vi "ArrayCharToString.vi"(7 "Type":T1(ring), 11 "TAB":string[][](array[string])) -> (3 "Instruction":string)   [LabVIEW 2020]
doc: "Convert array data to string instruction for script python"
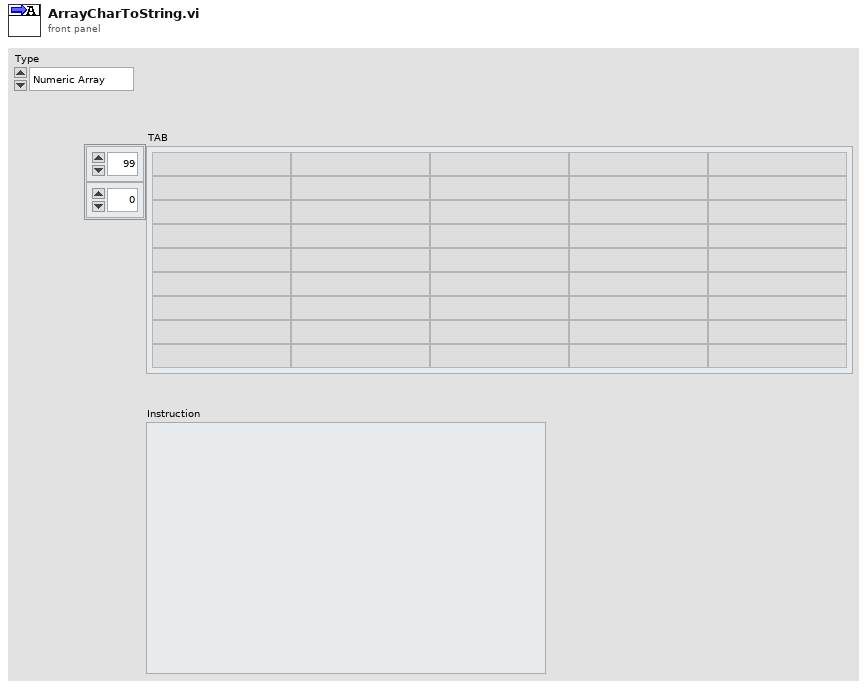
[diagram p1: front panel]
types:
  T1 = enum16{"Numeric Array", "String Array", "Sparse"}
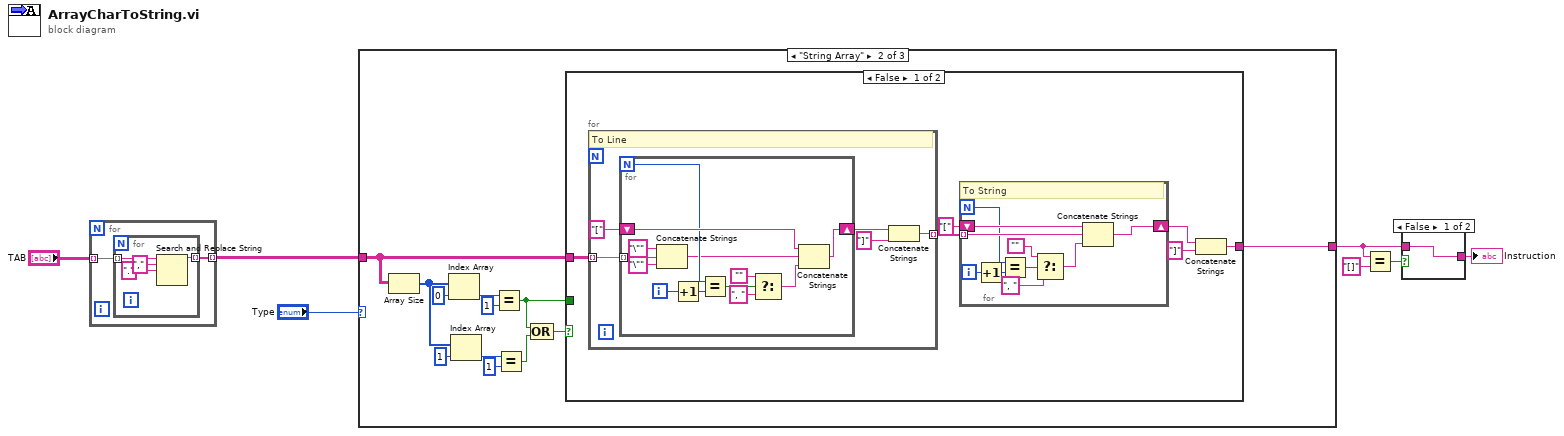
[diagram p0: block diagram]
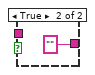
[diagram p2: hidden frame]
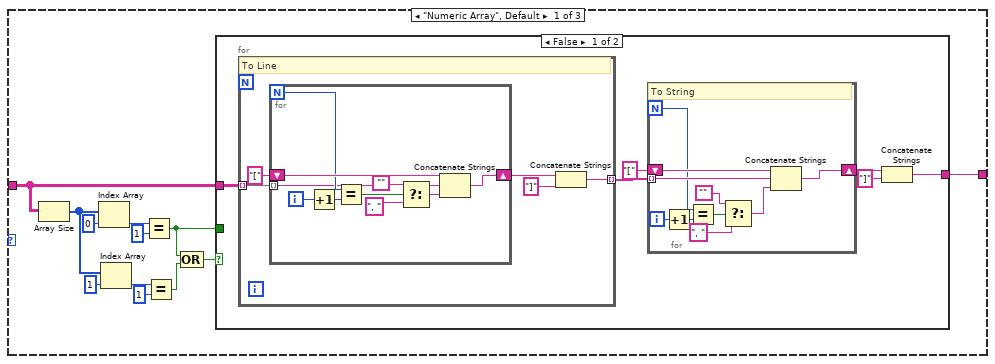
[diagram p3: hidden frame]
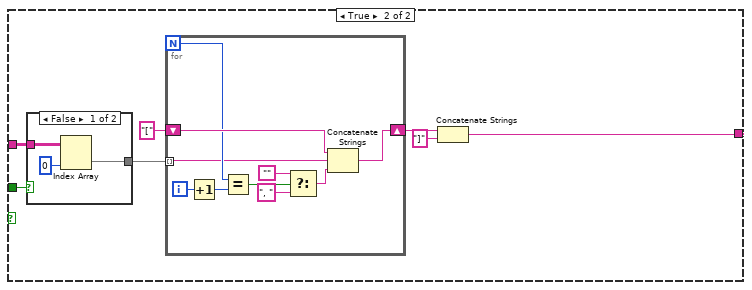
[diagram p4: hidden frame]
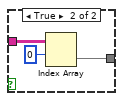
[diagram p5: hidden frame]
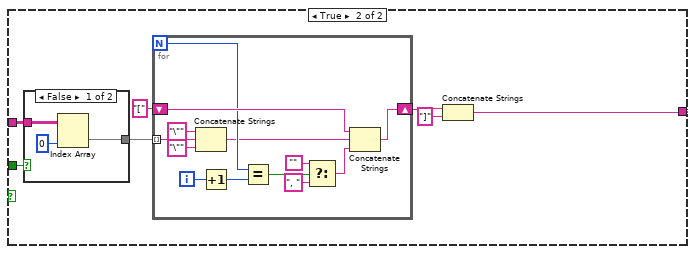
[diagram p6: hidden frame]
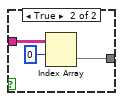
[diagram p7: hidden frame]
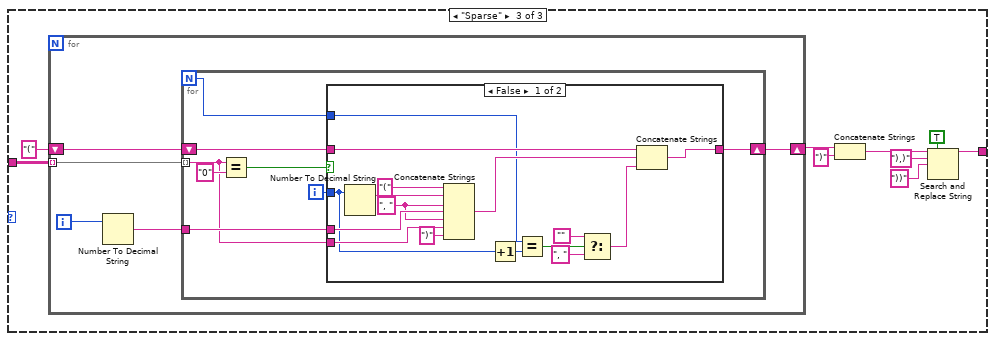
[diagram p8: hidden frame]
diagram:
  n1 = for {
    tunnel: "TAB" -> [w9] mode=indexing
    tunnel: [w8] -> w2 mode=indexing
    n2 = for {
      tunnel: w9 -> [w13] mode=indexing
      tunnel: [w10] -> w8 mode=indexing
      n3 = Search and Replace String(input string=w13, search string=",", replace string="." ("replace string (\"\")")) -> (result string=w10:string)  [unwired: 5 in, 3 out]
    }
  }
  n4 = case shown="\"String Array\"" "Type" {
    tunnel: w2 -> [w25 w91 w160]
    tunnel: [w22 w88 w155] -> w4
    frame "Numeric Array", Default {
      n5 = Array Size(array=w25) -> (size(s)=w20:i32[])
      n6 = Index Array(array=w20, index=0) -> (element=w19:i32)
      n7 = Index Array(array=w20, index=1) -> (element=w17:i32)
      n8 = Equal?(x=w19, y=1) -> (x = y?=w14:bool)
      n9 = Equal?(x=w17, y=1) -> (x = y?=w16:bool)
      n10 = Compound Arithmetic op=OR(w14, w16) -> (w15:bool)
      n11 = case shown="False" w15 {
        tunnel: [w27 w58] -> w22
        tunnel: w25 -> [w26 w60]
        tunnel: w14 -> [_ w57]
        frame False {
          n12 = for {
            tunnel: w26 -> [w46] mode=indexing
            tunnel: [w44] -> w31 mode=indexing
            # "To Line"
            n13 = for {
              N -> [w53]
              shift-right: [w55] -> w45
              shift-left: "[" ("t") -> [w56]
              tunnel: w46 -> [w47] mode=indexing
              i -> [w54]
              n14 = Increment(x=w54) -> (x+1=w52:i32)
              n15 = Equal?(x=w53, y=w52) -> (x = y?=w51:bool)
              n16 = Select(t="", s=w51, f=", ") -> (s? t:f=w49:string)
              n17 = Concatenate Strings(w56, w47, w49) -> (w55:string)
            }
            n18 = Concatenate Strings(w45, "]" ("t")) -> (w44:string)
          }
          n19 = for {
            N -> [w37]
            shift-right: [w39] -> w29
            shift-left: "[" -> [w41]
            tunnel: w31 -> [w40] mode=indexing
            i -> [w38]
            # "To String"
            n20 = Increment(x=w38) -> (x+1=w36:i32)
            n21 = Equal?(x=w37, y=w36) -> (x = y?=w35:bool)
            n22 = Select(t="", s=w35, f=", ") -> (s? t:f=w33:string)
            n23 = Concatenate Strings(w41, w40, w33) -> (w39:string)
          }
          n24 = Concatenate Strings(w29, "]" ("string")) -> (w27:string)
        }
        frame True {
          n25 = case shown="False" w57 {
            tunnel: w60 -> [w66 w69]
            tunnel: [w65 w68] -> w59
            frame False {
              n26 = Index Array(array=w66, index (col)=0 ("disabled index (col)")) -> (element=w65:string[])  [unwired: 1 in]
            }
            frame True {
              n27 = Index Array(array=w69, index (row)=0) -> (element=w68:string[])  [unwired: 1 in]
            }
          }
          n28 = for {
            N -> [w73]
            tunnel: w59 -> [w71] mode=indexing
            shift-right: [w70] -> w62
            shift-left: "[" -> [w79]
            i -> [w74]
            n29 = Increment(x=w74) -> (x+1=w78:i32)
            n30 = Equal?(x=w73, y=w78) -> (x = y?=w77:bool)
            n31 = Select(t="", s=w77, f=", ") -> (s? t:f=w72:string)
            n32 = Concatenate Strings(w79, w71, w72) -> (w70:string)
          }
          n33 = Concatenate Strings(w62, "]") -> (w58:string)
        }
      }
    }
    frame "String Array" {
      n34 = Array Size(array=w91) -> (size(s)=w86:i32[])
      n35 = Index Array(array=w86, index=0) -> (element=w85:i32)
      n36 = Index Array(array=w86, index=1) -> (element=w83:i32)
      n37 = Equal?(x=w85, y=1) -> (x = y?=w80:bool)
      n38 = Equal?(x=w83, y=1) -> (x = y?=w82:bool)
      n39 = Compound Arithmetic op=OR(w80, w82) -> (w81:bool)
      n40 = case shown="False" w81 {
        tunnel: [w93 w127] -> w88
        tunnel: w91 -> [w92 w129]
        tunnel: w80 -> [_ w126]
        frame False {
          n41 = for {
            tunnel: w92 -> [w112] mode=indexing
            tunnel: [w110] -> w97 mode=indexing
            # "To Line"
            n42 = for {
              N -> [w122]
              shift-right: [w124] -> w111
              shift-left: "[" ("t") -> [w125]
              tunnel: w112 -> [w115] mode=indexing
              i -> [w123]
              n43 = Concatenate Strings("\"" ("string"), w115, "\"" ("string")) -> (w116:string)
              n44 = Increment(x=w123) -> (x+1=w121:i32)
              n45 = Equal?(x=w122, y=w121) -> (x = y?=w120:bool)
              n46 = Select(t="", s=w120, f=", ") -> (s? t:f=w118:string)
              n47 = Concatenate Strings(w125, w116, w118) -> (w124:string)
            }
            n48 = Concatenate Strings(w111, "]" ("t")) -> (w110:string)
          }
          n49 = for {
            N -> [w103]
            shift-right: [w105] -> w95
            shift-left: "[" -> [w107]
            tunnel: w97 -> [w106] mode=indexing
            i -> [w104]
            # "To String"
            n50 = Increment(x=w104) -> (x+1=w102:i32)
            n51 = Equal?(x=w103, y=w102) -> (x = y?=w101:bool)
            n52 = Select(t="", s=w101, f=", ") -> (s? t:f=w99:string)
            n53 = Concatenate Strings(w107, w106, w99) -> (w105:string)
          }
          n54 = Concatenate Strings(w95, "]" ("string")) -> (w93:string)
        }
        frame True {
          n55 = case shown="False" w126 {
            tunnel: w129 -> [w135 w138]
            tunnel: [w134 w137] -> w128
            frame False {
              n56 = Index Array(array=w135, index (col)=0 ("disabled index (col)")) -> (element=w134:string[])  [unwired: 1 in]
            }
            frame True {
              n57 = Index Array(array=w138, index (row)=0) -> (element=w137:string[])  [unwired: 1 in]
            }
          }
          n58 = for {
            N -> [w145]
            tunnel: w128 -> [w143] mode=indexing
            shift-right: [w141] -> w131
            shift-left: "[" -> [w151]
            i -> [w146]
            n59 = Concatenate Strings("\"" ("string"), w143, "\"" ("string")) -> (w142:string)
            n60 = Increment(x=w146) -> (x+1=w150:i32)
            n61 = Equal?(x=w145, y=w150) -> (x = y?=w149:bool)
            n62 = Select(t="", s=w149, f=", ") -> (s? t:f=w144:string)
            n63 = Concatenate Strings(w151, w142, w144) -> (w141:string)
          }
          n64 = Concatenate Strings(w131, "]") -> (w127:string)
        }
      }
    }
    frame "Sparse" {
      n65 = for {
        tunnel: w160 -> [w163] mode=indexing
        shift-right: [w162] -> w158
        shift-left: "(" -> [w161]
        i -> [w165]
        n66 = Number To Decimal String(number=w165) -> (decimal integer string=w164:string)  [unwired: 1 in]
        n67 = for {
          N -> [w166]
          tunnel: w164 -> [w171]
          tunnel: w163 -> [w170] mode=indexing
          shift-right: [w167] -> w162
          shift-left: w161 -> [w168]
          i -> [w172]
          n68 = Equal?(x=w170, y="0") -> (x = y?=w169:bool)
          n69 = case shown="False" w169 {
            tunnel: w172 -> [w176 _]
            tunnel: w171 -> [w187 _]
            tunnel: w170 -> [w185 _]
            tunnel: w168 -> [w182 w190]
            tunnel: [w183 w190] -> w167
            tunnel: w166 -> [w175 _]
            frame False {
              w186 = ", " ("string")
              n70 = Number To Decimal String(number=w176) -> (decimal integer string=w188:string)  [unwired: 1 in]
              n71 = Concatenate Strings("(", w188, w186, w187, w186, w185, ")" ("string")) -> (w181:string)
              n72 = Increment(x=w176) -> (x+1=w180:i32)
              n73 = Equal?(x=w175, y=w180) -> (x = y?=w179:bool)
              n74 = Select(t="", s=w179, f=", ") -> (s? t:f=w174:string)
              n75 = Concatenate Strings(w182, w181, w174) -> (w183:string)
            }
            frame True {
            }
          }
        }
      }
      n76 = Concatenate Strings(w158, ")" ("string")) -> (w156:string)
      n77 = Search and Replace String(replace all?=TRUE ("replace all? (F)"), input string=w156, search string="),)", replace string="))" ("replace string (\"\")")) -> (result string=w155:string)  [unwired: 4 in, 3 out]
    }
  }
  n78 = Equal?(x=w4, y="[]") -> (x = y?=w6:bool)
  n79 = case shown="False" w6 {
    tunnel: [w191 ""] -> w5
    tunnel: w4 -> [w191 _]
    frame False {
    }
    frame True {
    }
  }
  "Instruction" <- w5
